vi "AdjustLeftRightSpeeds.vi"() -> ()   [LabVIEW 2017]
panel:
  out "Right":dbl
  out "Left":dbl
  in  "Trackwidth":dbl
  in  "Right":dbl
  in  "Left":dbl
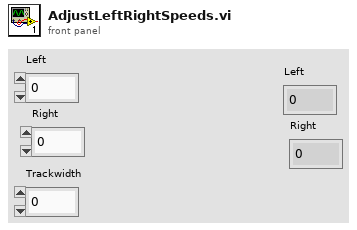
[diagram p1: front panel]
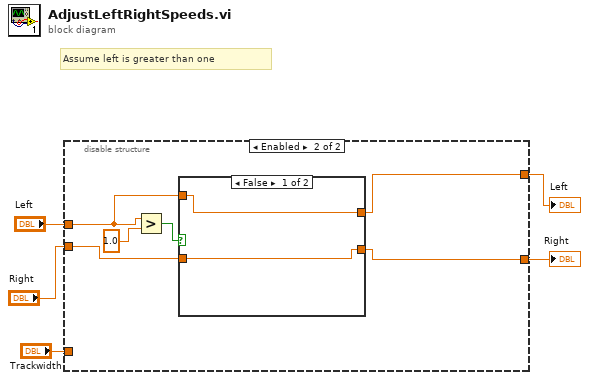
[diagram p0: block diagram]
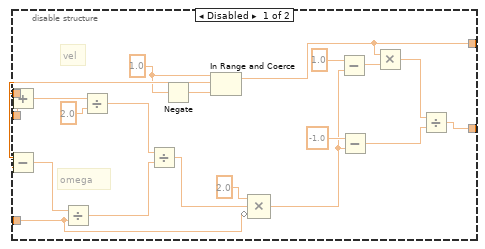
[diagram p2: hidden frame]
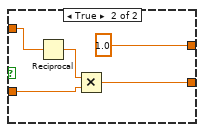
[diagram p3: hidden frame]
diagram:
  # "Assume left is greater than one"
  n1 = disable-structure shown="Enabled" {
    disable-tunnel: "Right" -> [w23 w28]
    disable-tunnel: "Left" -> [w21 w29]
    disable-tunnel: "Trackwidth" -> [w15 _]
    disable-tunnel: [w7 w26] -> w2
    disable-tunnel: [w6 w27] -> w1
    frame Disabled {
      w12 = 1.0 ("upper limit")
      # "omega"
      # "vel"
      n2 = Add(x=w21, y=w23) -> (x+y=w25:dbl)
      n3 = Subtract(x=w21, y=w23) -> (x-y=w22:dbl)
      n4 = Divide(x=w22, y=w15) -> (x/y=w17:dbl)
      n5 = Divide(x=w25, y=2.0) -> (x/y=w18:dbl)
      n6 = Divide(x=w18, y=w17) -> (x/y=w16:dbl)
      n7 = Negate(x=w12) -> (-x=w20:dbl)
      n8 = In Range and Coerce(upper limit=w12, x=w21, lower limit=w20) -> (coerced(x)=w7:dbl)  [unwired: 1 out]
      n9 = Compound Arithmetic op=MULTIPLY(2.0 ("value"), w16, invert w15) -> (w9:dbl)
      n10 = Subtract(x=1.0, y=w9) -> (x-y=w13:dbl)
      n11 = Subtract(x=-1.0, y=w9) -> (x-y=w8:dbl)
      n12 = Multiply(x=w7, y=w13) -> (x*y=w11:dbl)
      n13 = Divide(x=w11, y=w8) -> (x/y=w6:dbl)
    }
    frame Enabled {
      n14 = Greater?(x=w29, y=1.0) -> (0:w30:bool)
      n15 = case shown="False" w30 {
        tunnel: [w33 1.0 ("y")] -> w26
        tunnel: w29 -> [w33 w37]
        tunnel: w28 -> [w32 w35]
        tunnel: [w32 w34] -> w27
        frame False {
        }
        frame True {
          n16 = Reciprocal(x=w37) -> (1/x=w36:dbl)
          n17 = Multiply(x=w36, y=w35) -> (x*y=w34:dbl)
        }
      }
    }
  }
  "Left" <- w2
  "Right" <- w1
